vi "Write INodeFactory.vi"(10 "INodeFactory":refnum<class "INodeFactory.lvclass">, 11 "Project in":refnum<class "Project.lvclass">) -> (3 "Project out":refnum<class "Project.lvclass">)   [LabVIEW 2016, in "Project.lvclass"]
uses:
  Project.lvclass
  INodeFactory/INodeFactory.lvclass
  Project.lvclass/Project.ctl
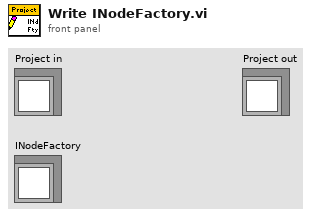
[diagram p1: front panel]
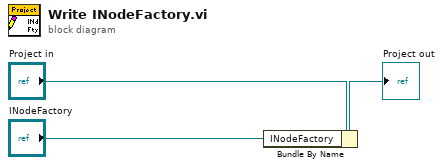
[diagram p0: block diagram]
diagram:
  n1 = Bundle By Name(cluster="Project in", "INodeFactory"="INodeFactory") -> (→"Project out":refnum<class "Project.lvclass">)
